vi "acquisition-running.vi"(3 "error in (no error)":errorcluster, 4 "Manufacturer":enum16{"Andor", "Xenics", "unknown"}(ring), 5 "xeva-camref-in":T2) -> (0 "error out":errorcluster, 1 "acquiring":bool, 2 "xeva-camref-out":T2)   [LabVIEW 2015]
uses:
  <vilib>/Xenics Infrared Solutions/Xeneth LabVIEW API/VIs/Controls/Camara.ctl
  <userlib>/atmcd32d.llb/Error Code Enum typedef.ctl
  <vilib>/Xenics Infrared Solutions/Xeneth LabVIEW API/Xeneth.lvlib
panel:
  out "andor-acquisition Status":T1=enum."DRV_NOT_INITIALIZED"
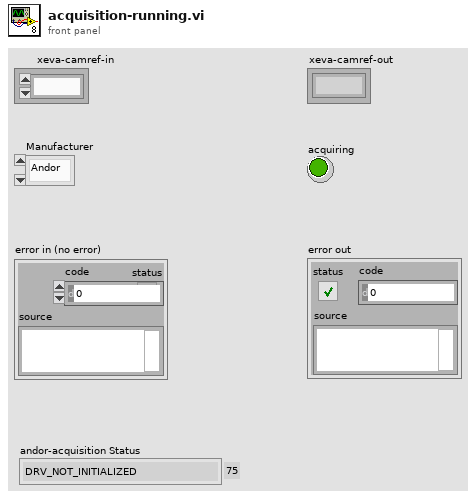
[diagram p1: front panel]
types:
  T1 = typedef "Error Code Enum typedef.ctl" = enum32{"N/A (0)", "DRV_ERROR_CODES", "DRV_SUCCESS", "DRV_VXDNOTINSTALLED", "DRV_ERROR_SCAN", "DRV_ERROR_CHECK_SUM", "DRV_ERROR_FILELOAD", "DRV_UNKNOWN_FUNC", "DRV_ERROR_VXD_INIT", "DRV_ERROR_ADDRESS", "DRV_ERROR_PAGELOCK", "DRV_ERROR_PAGEUNLOCK", "DRV_ERROR_BOARDTEST", "DRV_ERROR_ACK", "DRV_ERROR_UP_FIFO", "DRV_ERROR_PATTERN", "N/A (16)", "DRV_ACQUISITION_ERRORS", "DRV_ACQ_BUFFER", "DRV_ACQ_DOWNFIFO_FULL", "DRV_PROC_UNKONWN_INSTRUCTION", "DRV_ILLEGAL_OP_CODE", "DRV_KINETIC_TIME_NOT_MET", "DRV_ACCUM_TIME_NOT_MET", "DRV_NO_NEW_DATA", "N/A (25)", "DRV_SPOOLERROR", "N/A (27)", "N/A (28)", "N/A (29)", "N/A (30)", "N/A (31)", "N/A (32)", "DRV_TEMPERATURE_CODES", "DRV_TEMPERATURE_OFF", "DRV_TEMPERATURE_NOT_STABILIZED", "DRV_TEMPERATURE_STABILIZED", "DRV_TEMPERATURE_NOT_REACHED", "DRV_TEMPERATURE_OUT_RANGE", "DRV_TEMPERATURE_NOT_SUPPORTED", "DRV_TEMPERATURE_DRIFT", "N/A (41)", "N/A (42)", "N/A (43)", "N/A (44)", "N/A (45)", "N/A (46)", "N/A (47)", "N/A (48)", "DRV_GENERAL_ERRORS", "DRV_INVALID_AUX", "DRV_COF_NOTLOADED", "DRV_FPGAPROG", "DRV_FLEXERROR", "DRV_GPIBERROR", "N/A (55)", "N/A (56)", "N/A (57)", "N/A (58)", "N/A (59)", "N/A (60)", "N/A (61)", "N/A (62)", "N/A (63)", "DRV_DATATYPE", "DRV_DRIVER_ERRORS", "DRV_P1INVALID", "DRV_P2INVALID", "DRV_P3INVALID", "DRV_P4INVALID", "DRV_INIERROR", "DRV_COFERROR", "DRV_ACQUIRING", "DRV_IDLE", "DRV_TEMPCYCLE", "DRV_NOT_INITIALIZED", "DRV_P5INVALID", "DRV_P6INVALID", "DRV_INVALID_MODE", "DRV_INVALID_FILTER", "DRV_I2CERRORS", "DRV_I2CDEVNOTFOUND", "DRV_I2CTIMEOUT", "DRV_P7INVALID", "N/A (84)", "N/A (85)", "N/A (86)", "N/A (87)", "N/A (88)", "N/A (89)", "DRV_IOCERROR", "DRV_VRMVERSIONERROR"}
  T2 = typedef "Xeneth.lvlib/Camara.ctl" = refnum<k1>
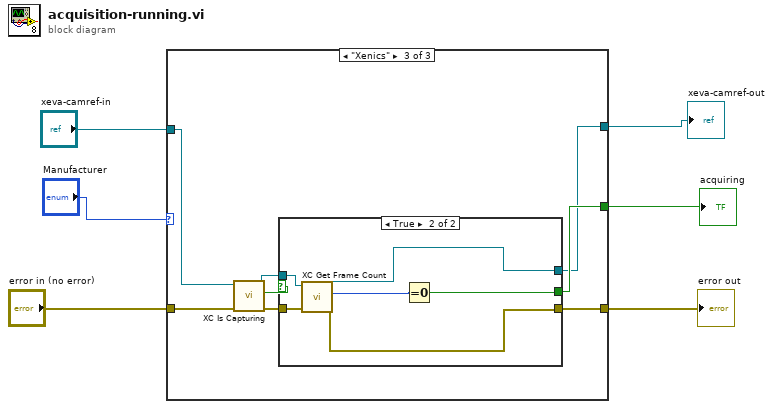
[diagram p0: block diagram]
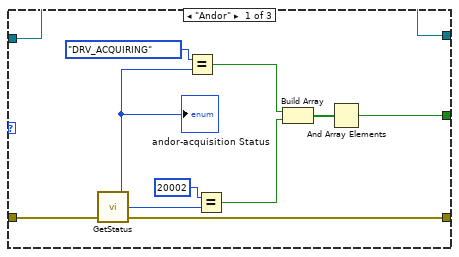
[diagram p2: hidden frame]
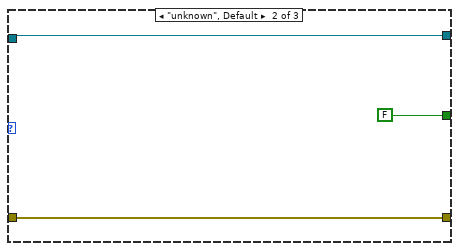
[diagram p3: hidden frame]
diagram:
  n1 = case shown="\"Xenics\"" "Manufacturer" {
    tunnel: [w8 FALSE w23] -> w5
    tunnel: [w15 w19 w21] -> w4
    tunnel: "error in (no error)" -> [w16 w19 w28]
    tunnel: "xeva-camref-in" -> [w7 w18 w27]
    tunnel: [w7 w18 w22] -> w1
    frame "Andor" {
      n2 = call <userlib>:"GetStatus.vi"("error in (no error)"=w16) -> ("error out"=w15:errorcluster, "DLL error code"=w13:u32, "status"=w14:T1)  [unwired: 2 in]
      "andor-acquisition Status" <- w14
      n3 = Equal?(x=Error_Code_Enum_typedef."DRV_ACQUIRING" ("Acquisition Status"), y=w14) -> (x = y?=w11:bool)
      n4 = Equal?(x=u32 20002 ("= temperature\naccepted"), y=w13) -> (x = y?=w10:bool)
      n5 = Build Array(w11, w10) -> (w9:bool[])
      n6 = And Array Elements(Boolean array=w9) -> (logical AND=w8:bool)
    }
    frame "unknown", Default {
    }
    frame "Xenics" {
      n7 = call <vilib>:"XC Is Capturing.vi"("error in (no error)"=w28, "Cam Ref"=w27) -> ("error out"=w26:errorcluster, "IsCapturing"=w25:bool, "Cam Ref Out"=w24:T2)  [unwired: 7 in]
      n8 = case shown="True" w25 {
        selector: w25 -> [w29 _]
        tunnel: w26 -> [w30 w37]
        tunnel: w24 -> [w31 w36]
        tunnel: [w29 w32] -> w23
        tunnel: [w31 w35] -> w22
        tunnel: [w30 w34] -> w21
        frame False {
        }
        frame True {
          n9 = call <vilib>:"XC Get Frame Count.vi"("error in (no error)"=w37, "Cam Ref"=w36) -> ("error out"=w34:errorcluster, "Frame Count"=w33:u32, "Cam Ref Out"=w35:T2)  [unwired: 7 in]
          n10 = Equal To 0?(x=w33) -> (x = 0?=w32:bool)
        }
      }
    }
  }
  "acquiring" <- w5
  "error out" <- w4
  "xeva-camref-out" <- w1
